vi "quaternion_multiply.vi"(8 "q2":dbl[](array[numeric]), 11 "q1":dbl[](array[numeric])) -> (3 "q1 * q2":dbl[](array[numeric]))   [LabVIEW 2012]
panel:
  # "Multiply two quaternions."
  # "w"
  # "x1"
  # "x2"
  # "x3"
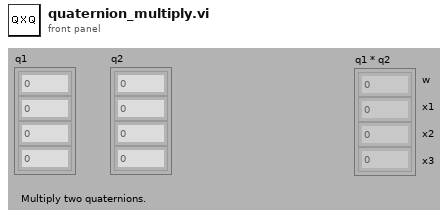
[diagram p1: front panel]
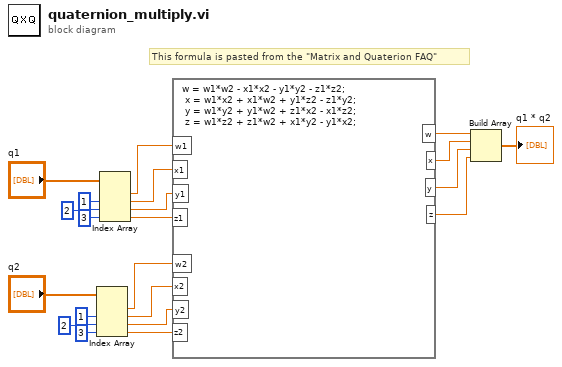
[diagram p0: block diagram]
diagram:
  # "This formula is pasted from the \"Matrix and Quaterion FAQ\""
  n1 = Index Array(array="q2", index #2=1 ("index"), index #3=2 ("index"), index #4=3 ("index")) -> (element #1=w13:dbl, element #2=w12:dbl, element #3=w11:dbl, element #4=w10:dbl)  [unwired: 1 in]
  n2 = Index Array(array="q1", index #2=1 ("index"), index #3=2 ("index"), index #4=3 ("index")) -> (element #1=w6:dbl, element #2=w7:dbl, element #3=w8:dbl, element #4=w9:dbl)  [unwired: 1 in]
  n3 = formula code="w = w1*w2 - x1*x2 - y1*y2 - z1*z2;\n\tx = w1*x2 + x1*w2 + y1*z2 - z1*y2;\n\ty = w1*y2 + y1*w2 + z1*x2 - x1*z2;\n\tz = w1*z2 + z1*w2 + x1*y2 - y1*x2;"("w1"=w6, "x1"=w7, "y1"=w8, "z1"=w9, "w2"=w13, "x2"=w12, "y2"=w11, "z2"=w10) -> ("w"=w5:dbl, "x"=w4:dbl, "y"=w3:dbl, "z"=w2:dbl)
  n4 = Build Array(w5, w4, w3, w2) -> (→"q1 * q2":dbl[])
